vi "target_b2g1.vi"   [LabVIEW 2011]
uses:
  Output - Cluster b2g1.ctl
  Input - Cluster b2g1.ctl
  <vilib>/Platform/TimedLoop/XDataNode/timing_clust.ctl
  <vilib>/Platform/TimedLoop/XDataNode/nitl_modes.ctl
  <vilib>/Platform/TimedLoop/XDataNode/wakeup.ctl
  <vilib>/Platform/TimedLoop/XDataNode/XDataNode.xnode
  <vilib>/Platform/TimedLoop/XDataNode/XDNodeRunTimeDep.lvlib
panel:
  # "The Network Variable Engine and Variable Client Support must be installed on the RT target\nfor this application to function properly. If the Network Variable Engine is not supported on\nthe target (e.g.  FP-2000 with <32MB of RAM), open the project and move the variable library\nto My Computer in the project. Doing this will deploy the variables to localhost but\nwill still require that Variable Client Support be installed on the RT target."
types:
  T1 = typedef "XDNodeRunTimeDep.lvlib/timing_clust.ctl" = cluster{"Expected End [f-1]":u64, "Actual End [f-1]":u64, "Finished Late? [f-1]":bool, "Expected End [i-1]":u64, "Actual End [i-1]":u64, "Finished Late? [i-1]":bool, "Expected Start [i]":u64, "Actual Start [i]":u64, "Expected Start [f]":u64, "Actual Start [f]":u64, "Source Name":string, "Structure Name":string, "Period":i64, "Deadline":i64, "Offset":i64, "Start":i64, "Priority":i32, "Timeout":i32, "Mode":T2, "Wakeup Reason":T3, "Error":errorcluster, "Source Type":string, "Secondary Source Type":string, "Global End Time":u64, "Global Start Time":u64, "Frame Duration":u64, "Iteration Duration":u64, "Assigned CPU":i32, "I/O Scan Engine Mode":u32}
  T2 = typedef "XDNodeRunTimeDep.lvlib/nitl_modes.ctl" = enum32{"No Change", "Process missed periods, maintain original phase", "Discard missed periods, maintain original phase", "Process missed periods, ignore original phase", "Discard missed periods, ignore original phase"}
  T3 = typedef "XDNodeRunTimeDep.lvlib/wakeup.ctl" = enum32{"Normal", "Aborted", "Asynchronous wakeup", "Timing source error", "Timed loop error", "Timeout"}
  T4 = typedef "Output - Cluster b2g1.ctl" = cluster{"DFS-1 [dl]":u64, "FS-3 [l]":dbl, "DFS-1 [l/min]":dbl, "DS-1 [bar]":dbl, "V-10 ZU":bool, "V-14 ZU":bool, "FS-1 [l]":dbl, "FS-2 [l]":dbl, "TS-4 [°C]":dbl, "HS-1":bool, "V-13 [%]":u8, "V-15 [%]":u8, "P-4 [%]":u8, "P-5 [%]":u8, "Dosierung":bool, "MR Max Füllstand":bool, "MR Min Füllstand":bool, "Dosiermenge [l]":sgl, "V-14 AUF":bool, "V-10 AUF":bool, "T-1 Max Füllstand":bool, "T-1 Min Füllstand":bool, "T-2 Max Füllstand":bool, "T-2 Min Füllstand":bool, "pHS-1 [pH]":dbl, "P-4 RUN":bool, "P-5 RUN ":bool, "V-33 AUF":bool, "V-33 ZU":bool, "V-34 AUF":bool, "V-34 ZU":bool, "P-4 ERR":bool, "P-5 ERR":bool, "TS-5 [°C]":dbl, "GZ-1 [dl]":u64, "TS-6 [°C]":dbl, "DS-3 [bar]":dbl, "P-9 RUN":bool}
  T5 = typedef "Input - Cluster b2g1.ctl" = cluster{"V-13 [%]":u8, "V-15 [%]":u8, "Log-Target":bool, "P-4":bool, "P-4 Drehzahl [%]":u8, "Temperaturregelung":bool, "Überdruckregelung":bool, "Füllstandsregulierung":bool, "V-10":bool, "Log-Host":bool, "V-14":bool, "P-5":bool, "P-5 Drehzahl [%]":u8, "HS-1":bool, "Füllstand  P":sgl, "Füllstand I":sgl, "Füllstand D":sgl, "Füllstand Soll [l]":sgl, "Druck  P":sgl, "Druck I":sgl, "Druck D":sgl, "Druck Soll [bar]":sgl, "Temp Soll [°C]":sgl, "Dosierung":bool, "Dosiermenge [l]":sgl, "Dosiergeschw. [l/min]":sgl, "Tank":bool, "Hysterese [°C]":sgl, "MR Füllstandsüberwachung":bool, "Tank Füllstandsüberwachung":bool, "Log Target [ms]":u32, "Log Host [s]":u32, "P-5 EIN [min]":u8, "P-5 AUS [min]":u8, "Zirkulation":bool, "V-33":bool, "V-34":bool, "P-9":bool}
  T6 = cluster{"Durchflussregelung":dbl, "Temperaturregelung":bool, "STOP":bool, "Zirkulation":u64, "Dosierung Zeit":u64}
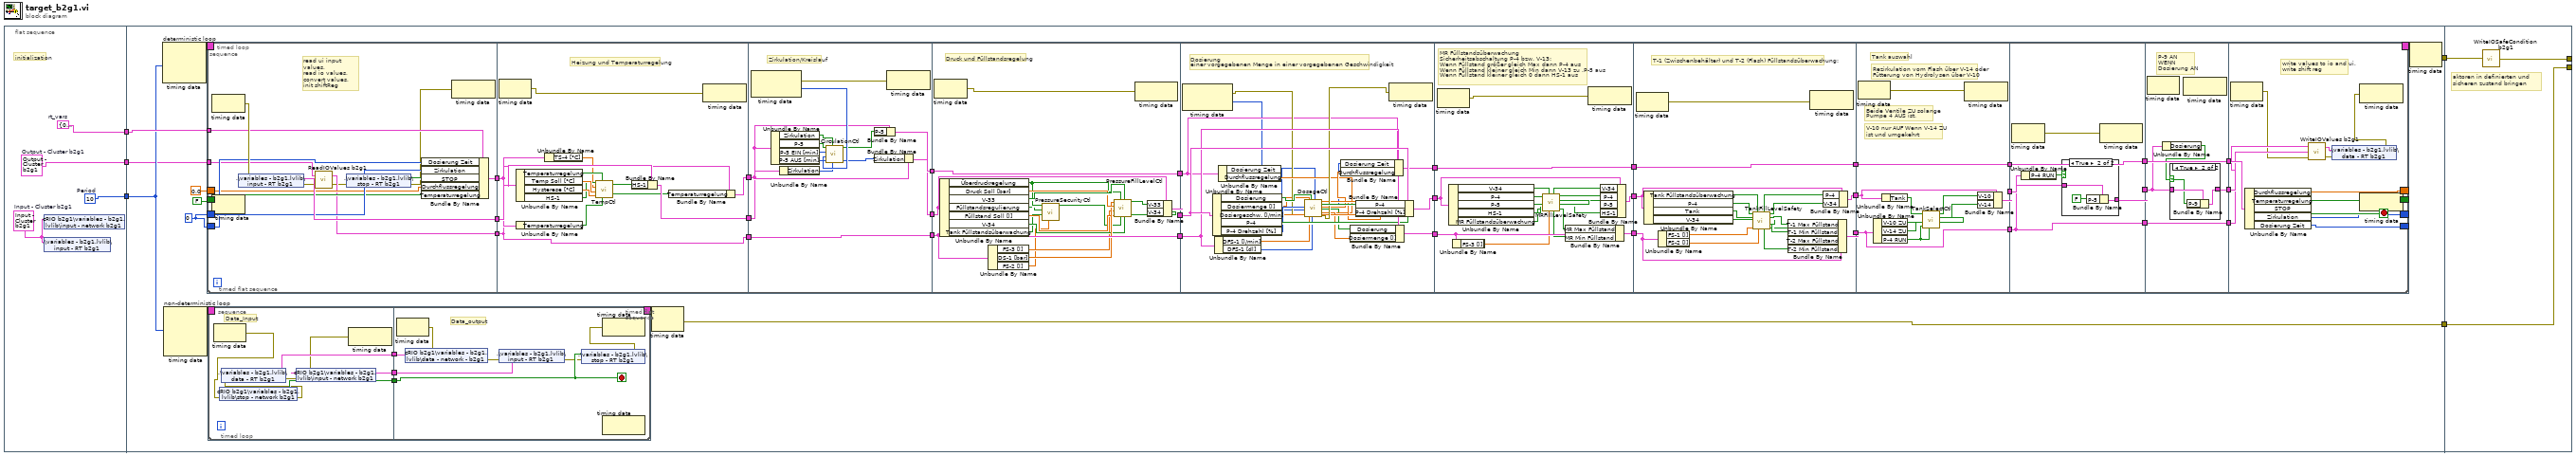
[diagram p0: block diagram]
diagram:
  n1 = flat-sequence {
    tunnel: [w9] -> w5
    tunnel: [w8] -> w4
    tunnel: [w6] -> w3
    tunnel: w5 -> [w15]
    tunnel: w4 -> [w14]
    tunnel: w3 -> [w13]
    tunnel: [w12] -> w2
    tunnel: [w11] -> w1
    tunnel: w2 -> [w329]
    tunnel: w1 -> [w331]
    tunnel: [w330] -> _
    tunnel: [w329] -> _
    frame #0 {
      w6 = T4 {"DFS-1 [dl]"=0, "FS-3 [l]"=0.0, "DFS-1 [l/min]"=0.0, "DS-1 [bar]"=0.0, "V-10 ZU"=FALSE, "V-14 ZU"=FALSE, "FS-1 [l]"=0.0, "FS-2 [l]"=0.0, "TS-4 [°C]"=0.0, "HS-1"=FALSE, "V-13 [%]"=0, "V-15 [%]"=0, "P-4 [%]"=0, "P-5 [%]"=0, "Dosierung"=FALSE, "MR Max Füllstand"=FALSE, "MR Min Füllstand"=FALSE, "Dosiermenge [l]"=0.0, "V-14 AUF"=FALSE, "V-10 AUF"=FALSE, "T-1 Max Füllstand"=FALSE, "T-1 Min Füllstand"=FALSE, "T-2 Max Füllstand"=FALSE, "T-2 Min Füllstand"=FALSE, "pHS-1 [pH]"=0.0, "P-4 RUN"=FALSE, "P-5 RUN "=FALSE, "V-33 AUF"=FALSE, "V-33 ZU"=FALSE, "V-34 AUF"=FALSE, "V-34 ZU"=FALSE, "P-4 ERR"=FALSE, "P-5 ERR"=FALSE, "TS-5 [°C]"=0.0, "GZ-1 [dl]"=0, "TS-6 [°C]"=0.0, "DS-3 [bar]"=0.0, "P-9 RUN"=FALSE}  # Output - Cluster b2g1
      w7 = T5 {"V-13 [%]"=0, "V-15 [%]"=0, "Log-Target"=FALSE, "P-4"=FALSE, "P-4 Drehzahl [%]"=0, "Temperaturregelung"=FALSE, "Überdruckregelung"=FALSE, "Füllstandsregulierung"=FALSE, "V-10"=FALSE, "Log-Host"=FALSE, "V-14"=FALSE, "P-5"=FALSE, "P-5 Drehzahl [%]"=0, "HS-1"=FALSE, "Füllstand  P"=0.0, "Füllstand I"=0.0, "Füllstand D"=0.0, "Füllstand Soll [l]"=0.0, "Druck  P"=0.0, "Druck I"=0.0, "Druck D"=0.0, "Druck Soll [bar]"=0.0, "Temp Soll [°C]"=0.0, "Dosierung"=FALSE, "Dosiermenge [l]"=0.0, "Dosiergeschw. [l/min]"=0.0, "Tank"=FALSE, "Hysterese [°C]"=0.0, "MR Füllstandsüberwachung"=FALSE, "Tank Füllstandsüberwachung"=FALSE, "Log Target [ms]"=0, "Log Host [s]"=0, "P-5 EIN [min]"=0, "P-5 AUS [min]"=0, "Zirkulation"=FALSE, "V-33"=FALSE, "V-34"=FALSE, "P-9"=FALSE}  # Input - Cluster b2g1
      w9 = T6 {"Durchflussregelung"=0.0, "Temperaturregelung"=FALSE, "STOP"=FALSE, "Zirkulation"=0, "Dosierung Zeit"=0}  # rt_vars
      w8 = i64 10  # Period
      # "initialization"
      n2 = shared-variable "cRIO b2g1\\variables - b2g1.lvlib\\input - network b2g1"(w7) -> ()  [unwired: 1 in, 1 out]
      n3 = shared-variable ".\\variables - b2g1.lvlib\\input - RT b2g1"(w7) -> ()  [unwired: 1 in, 1 out]
    }
    frame #1 {
      w10 = u64 0
      n4 = node-c288 ("Input Node")(w14) -> (w21:T1)  [unwired: 2 in]
      n5 = node-c288 ("Input Node")(w14) -> (w19:T1)  [unwired: 3 in]
      n6 = timed-loop "deterministic loop" {
        timing: w21 -> [_]
        timing-out: [_] -> w20
        shift-right: [w65] -> _
        shift-left: 0.0 -> [w64]
        shift-right: [w63] -> _
        shift-left: FALSE ("Temperaturregelung") -> [w61]
        tunnel: w15 -> [w62]
        tunnel: w13 -> [w60]
        shift-right: [w59] -> _
        shift-left: w10 -> [w58]
        shift-right: [w57] -> _
        shift-left: w10 -> [w56]
        stop <- w312 stop-if-true
        n7 = timed-sequence {
          timing: _ -> [_]
          timing-out: _ -> [_]
          tunnel: [w103] -> w65
          tunnel: w64 -> [w102]
          tunnel: [w99] -> w63
          tunnel: w62 -> [w98]
          tunnel: w61 -> [w96]
          tunnel: w60 -> [w91]
          tunnel: [w78] -> w59
          tunnel: w58 -> [w77]
          tunnel: [w73] -> w57
          tunnel: w56 -> [w72]
          n8 = timed-flat-sequence {
            tunnel: [w119] -> w101
            tunnel: [w109] -> w100
            tunnel: w102 -> [w112]
            tunnel: w98 -> [w117]
            tunnel: [w116] -> w97
            tunnel: w96 -> [w111]
            tunnel: w91 -> [w110]
            tunnel: w77 -> [w115]
            tunnel: w72 -> [w114]
            tunnel: w101 -> [w134]
            tunnel: w100 -> [w126]
            tunnel: [w126] -> w84
            tunnel: w97 -> [w130]
            tunnel: [w131] -> w82
            tunnel: [w133] -> w80
            tunnel: w84 -> [w156]
            tunnel: [w156] -> w83
            tunnel: w82 -> [w149]
            tunnel: [w150] -> w81
            tunnel: w80 -> [w147]
            tunnel: [w148] -> w79
            tunnel: [w179] -> w105
            tunnel: w83 -> [w177]
            tunnel: [w177] -> w104
            tunnel: w81 -> [w181]
            tunnel: [w181] -> w95
            tunnel: w79 -> [w178]
            tunnel: w105 -> [w210]
            tunnel: [w208] -> w90
            tunnel: w104 -> [w209]
            tunnel: [w203] -> w89
            tunnel: w95 -> [w195]
            tunnel: [w199] -> w88
            tunnel: w90 -> [w223]
            tunnel: [w222] -> w94
            tunnel: w89 -> [w232]
            tunnel: [w231] -> w93
            tunnel: w88 -> [w234]
            tunnel: [w234] -> w92
            tunnel: w94 -> [w244]
            tunnel: [w245] -> w87
            tunnel: w93 -> [w255]
            tunnel: [w254] -> w86
            tunnel: w92 -> [w257]
            tunnel: [w257] -> w85
            tunnel: w87 -> [w266]
            tunnel: [w267] -> w76
            tunnel: w86 -> [w270]
            tunnel: [w270] -> w75
            tunnel: w85 -> [w273]
            tunnel: [w273] -> w74
            tunnel: w76 -> [w282]
            tunnel: [w281] -> w71
            tunnel: w75 -> [w280]
            tunnel: [w280] -> w69
            tunnel: w74 -> [w284]
            tunnel: [w284] -> w67
            tunnel: w71 -> [w295]
            tunnel: [w296] -> w70
            tunnel: w69 -> [w298]
            tunnel: [w298] -> w68
            tunnel: w67 -> [w297]
            tunnel: [w297] -> w66
            tunnel: w70 -> [w309]
            tunnel: w68 -> [w308]
            tunnel: [w313] -> w103
            tunnel: [w314] -> w99
            tunnel: w66 -> [w315]
            tunnel: [w311] -> w78
            tunnel: [w310] -> w73
            frame #0 {
              # "read ui input values,\nread io values,\nconvert values,\ninit shiftReg"
              n9 = node-c288 ("Output Node")() -> (w118:errorcluster)  [unwired: 1 in]
              n10 = shared-variable ".\\variables - b2g1.lvlib\\input - RT b2g1"(error in=w118) -> (w119:T5, error out=w108:errorcluster)
              n11 = call "ReadIOValues b2g1.vi"("error in"=w108, "Output - Cluster b2g1 2"=w110) -> ("error out"=w107:errorcluster, "Output - Cluster b2g1"=w109:T4)
              n12 = shared-variable ".\\variables - b2g1.lvlib\\stop - RT b2g1"(error in=w107) -> (w113:bool, error out=w106:errorcluster)
              n13 = Bundle By Name(cluster=w117, "Dosierung Zeit"=w114, "Zirkulation"=w115, "STOP"=w113, "Durchflussregelung"=w112, "Temperaturregelung"=w111) -> (w116:T6)
              n14 = node-c288 ("Input Node")(w106) -> ()  [unwired: 1 out]
            }
            frame #1 {
              # "Heizung und Temperaturregelung"
              n15 = node-c288() -> (w138:errorcluster)  [unwired: 1 in]
              n16 = Unbundle By Name(w134) -> ("Temperaturregelung"=w137:bool, "Temp Soll [°C]"=w136:sgl, "Hysterese [°C]"=w135:sgl, "HS-1"=w127:bool)
              n17 = Unbundle By Name(w130) -> ("Temperaturregelung"=w129:bool)
              n18 = Unbundle By Name(w126) -> ("TS-4 [°C]"=w125:dbl)
              n19 = call "TempCtl.vi"("shiftReg"=w129, "enable"=w137, "Hysterese"=w135, "Soll"=w136, "IST"=w125, "heating"=w127) -> ("shiftReg"=w128:bool, "heating"=w132:bool)
              n20 = Bundle By Name(cluster=w134, "HS-1"=w132) -> (w133:T5)
              n21 = Bundle By Name(cluster=w130, "Temperaturregelung"=w128) -> (w131:T6)
              n22 = node-c288(w138) -> ()  [unwired: 1 out]
            }
            frame #2 {
              # "Zirkulation/Kreislauf"
              n23 = node-c288() -> (w157:errorcluster, w155:i64)  [unwired: 1 in]
              n24 = Unbundle By Name(w147) -> ("Zirkulation"=w152:bool, "P-5"=w151:bool, "P-5 EIN [min]"=w154:u8, "P-5 AUS [min]"=w153:u8)
              n25 = Unbundle By Name(w149) -> ("Zirkulation"=w144:u64)
              n26 = call "CirculationCtl.vi"("shiftReg[ms]"=w144, "enable"=w152, "Actual Start [ms]"=w155, "OffTime [min]"=w153, "OnTime [min]"=w154, "Pump"=w151) -> ("shiftReg[ms]"=w145:u64, "Pump"=w146:bool)  [unwired: 3 in, 1 out]
              n27 = Bundle By Name(cluster=w147, "P-5"=w146) -> (w148:T5)
              n28 = Bundle By Name(cluster=w149, "Zirkulation"=w145) -> (w150:T6)
              n29 = node-c288(w157) -> ()  [unwired: 1 out]
            }
            frame #3 {
              # "Druck und Füllstandsregelung"
              n30 = node-c288() -> (w180:errorcluster)  [unwired: 1 in]
              n31 = Unbundle By Name(w178) -> ("Überdruckregelung"=w167:bool, "Druck Soll [bar]"=w175:sgl, "V-33"=w176:bool, "Füllstandsregulierung"=w166:bool, "Füllstand Soll [l]"=w172:sgl, "V-34"=w173:bool, "Tank Füllstandsüberwachung"=w165:bool)
              n32 = Unbundle By Name(w177) -> ("FS-3 [l]"=w171:dbl, "DS-1 [bar]"=w174:dbl, "FS-2 [l]"=w168:dbl)
              n33 = call "PressureSecurityCtl.vi"("FS-2 [l]"=w168, "Tank Füllstandsüberwachung"=w165, "Füllstandsregulierung"=w166, "Überdruckregelung"=w167) -> ("Füllstandsregulierung"=w164:bool)  [unwired: 7 in]
              n34 = call "PressureFillLevelCtl.vi"("LiquidValve"=w173, "GasValve"=w176, "FillLevelCtl"=w164, "PressureCtl"=w167, "V_setpoint"=w172, "V_value"=w171, "P_setpoint"=w175, "P_value"=w174) -> ("LiquidValve"=w169:bool, "GasValve"=w170:bool)  [unwired: 2 in]
              n35 = node-c288(w180) -> ()  [unwired: 1 out]
              n36 = Bundle By Name(cluster=w178, "V-33"=w170, "V-34"=w169) -> (w179:T5)
            }
            frame #4 {
              # "Dosierung \neiner vorgegebenen Menge in einer vorgegebenen Geschwindigkeit"
              n37 = node-c288() -> (w196:errorcluster, w190:i64)  [unwired: 1 in]
              n38 = Unbundle By Name(w210) -> ("Dosierung"=w201:bool, "Dosiermenge [l]"=w187:sgl, "Dosiergeschw. [l/min]"=w204:sgl, "P-4"=w207:bool, "P-4 Drehzahl [%]"=w206:u8)
              n39 = Unbundle By Name(w209) -> ("DFS-1 [l/min]"=w192:dbl, "DFS-1 [dl]"=w193:u64)
              n40 = Unbundle By Name(w195) -> ("Dosierung Zeit"=w191:u64, "Durchflussregelung"=w197:dbl)
              n41 = call "DosageCtl.vi"("setpoint volume flow [l/min]"=w204, "pump"=w207, "value speed [%]"=w206, "shiftReg int"=w191, "shiftReg dbl"=w197, "error in (no error)"=w196, "setpoint volume [l]"=w187, "value volume flow [l/min]"=w192, "enable"=w201, "value volume [dl]"=w193, "Actual Start [f]"=w190) -> ("pump"=w194:bool, "speed [%]"=w202:dbl, "shiftReg int"=w189:u64, "shiftreg dbl"=w198:dbl, "enable"=w188:bool, "volume[l]"=w200:dbl, "error out"=w205:errorcluster)  [unwired: 2 in]
              n42 = Bundle By Name(cluster=w195, "Dosierung Zeit"=w189, "Durchflussregelung"=w198) -> (w199:T6)
              n43 = Bundle By Name(cluster=w209, "Dosierung"=w188, "Dosiermenge [l]"=w200) -> (w203:T4)
              n44 = Bundle By Name(cluster=w210, "P-4"=w194, "P-4 Drehzahl [%]"=w202) -> (w208:T5)
              n45 = node-c288(w205) -> ()  [unwired: 1 out]
            }
            frame #5 {
              # "MR Füllstandsüberwachung\nSicherheitsabschaltung P-4 bzw. V-13:\nWenn Füllstand größer gleich Max dann P-4 aus\nWenn Füllstand kleiner gleich Min dann V-13 zu ,P-5 aus\nWenn Füllstand kleiner gleich 0 dann HS-1 aus"
              n46 = node-c288() -> (w233:errorcluster)  [unwired: 1 in]
              n47 = Unbundle By Name(w223) -> ("V-34"=w227:bool, "P-4"=w226:bool, "P-5"=w225:bool, "HS-1"=w224:bool, "MR Füllstandsüberwachung"=w217:bool)
              n48 = Unbundle By Name(w232) -> ("FS-3 [l]"=w228:dbl)
              n49 = call "MRFillLevelSafety.vi"("fill level [l]"=w228, "Valve"=w227, "enable"=w217, "Heating"=w224, "Circulation"=w225, "Pump"=w226) -> ("max level"=w230:bool, "Heating"=w218:bool, "Circulation"=w219:bool, "Pump"=w220:bool, "min level"=w229:bool, "Valve"=w221:bool)
              n50 = Bundle By Name(cluster=w232, "MR Max Füllstand"=w230, "MR Min Füllstand"=w229) -> (w231:T4)
              n51 = node-c288(w233) -> ()  [unwired: 1 out]
              n52 = Bundle By Name(cluster=w223, "V-34"=w221, "P-4"=w220, "P-5"=w219, "HS-1"=w218) -> (w222:T5)
            }
            frame #6 {
              # "T-1 (Zwischenbehälter) und T-2 (Flash) Füllstandsüberwachung:"
              n53 = node-c288() -> (w256:errorcluster)  [unwired: 1 in]
              n54 = Unbundle By Name(w244) -> ("Tank Füllstandsüberwachung"=w240:bool, "P-4"=w243:bool, "Tank"=w241:bool, "V-34"=w242:bool)
              n55 = Unbundle By Name(w255) -> ("FS-1 [l]"=w249:dbl, "FS-2 [l]"=w251:dbl)
              n56 = call "TankFillLevelSafety.vi"("pump"=w243, "enable"=w240, "tank"=w241, "outlet valve"=w242, "fill level t-1"=w249, "fill level t-2"=w251) -> ("pump"=w247:bool, "outlet valve"=w246:bool, "max level t-1"=w248:bool, "min level t-1"=w253:bool, "min level t-2"=w252:bool, "max level t-2"=w250:bool)  [unwired: 3 in, 1 out]
              n57 = Bundle By Name(cluster=w255, "T-1 Max Füllstand"=w248, "T-1 Min Füllstand"=w253, "T-2 Max Füllstand"=w250, "T-2 Min Füllstand"=w252) -> (w254:T4)
              n58 = node-c288(w256) -> ()  [unwired: 1 out]
              n59 = Bundle By Name(cluster=w244, "P-4"=w247, "V-34"=w246) -> (w245:T5)
            }
            frame #7 {
              # "V-10 nur AUF Wenn V-14 ZU\nist und umgekehrt"
              # "Beide Ventile ZU solange \nPumpe 4 AUS ist."
              # "Rezirkulation vom Flash über V-14 oder \nFütterung von Hydrolysen über V-10"
              # "Tank auswahl"
              n60 = node-c288() -> (w271:errorcluster)  [unwired: 1 in]
              n61 = Unbundle By Name(w270) -> ("V-10 ZU"=w268:bool, "V-14 ZU"=w269:bool, "P-4 RUN"=w263:bool)
              n62 = Unbundle By Name(w266) -> ("Tank"=w272:bool)
              n63 = call "TankSelectCtl.vi"("pump"=w263, "enable"=w263, "valve t-2 close"=w269, "valve t-1 close"=w268, "Tank"=w272) -> ("valve t-2"=w264:bool, "valve t-1"=w265:bool)  [unwired: 5 in]
              n64 = node-c288(w271) -> ()  [unwired: 1 out]
              n65 = Bundle By Name(cluster=w266, "V-10"=w265, "V-14"=w264) -> (w267:T5)
            }
            frame #8 {
              n66 = node-c288() -> (w283:errorcluster)  [unwired: 1 in]
              n67 = Unbundle By Name(w280) -> ("P-4 RUN"=w279:bool)
              n68 = case shown="True" w279 {
                tunnel: w282 -> [w285 w288]
                tunnel: [w285 w287] -> w281
                frame False {
                }
                frame True {
                  n69 = Bundle By Name(cluster=w288, "P-5"=FALSE) -> (w287:T5)
                }
              }
              n70 = node-c288(w283) -> ()  [unwired: 1 out]
            }
            frame #9 {
              # "P-9 AN\nWENN \nDosierung AN"
              n71 = node-c288() -> ()  [unwired: 1 in, 1 out]
              n72 = Unbundle By Name(w295) -> ("Dosierung"=w294:bool)
              n73 = case shown="True" w294 {
                selector: w294 -> [_ w300]
                tunnel: w295 -> [w299 w302]
                tunnel: [w299 w301] -> w296
                frame False {
                }
                frame True {
                  n74 = Bundle By Name(cluster=w302, "P-9"=w300) -> (w301:T5)
                }
              }
              n75 = node-c288() -> ()  [unwired: 1 in, 1 out]
            }
            frame #10 {
              # "write values to io and ui,\nwrite shift reg"
              n76 = node-c288() -> (w306:errorcluster)  [unwired: 1 in]
              n77 = Unbundle By Name(w315) -> ("Durchflussregelung"=w313:dbl, "Temperaturregelung"=w314:bool, "STOP"=w312:bool, "Zirkulation"=w311:u64, "Dosierung Zeit"=w310:u64)
              n78 = call "WriteIOValues b2g1.vi"("error in"=w306, "Output - Cluster b2g1"=w308, "input cluster"=w309) -> ("error out"=w305:errorcluster, "output cluster"=w307:T4)
              n79 = shared-variable ".\\variables - b2g1.lvlib\\data - RT b2g1"(w307, error in=w305) -> (error out=w316:errorcluster)
              n80 = node-c288(w316) -> ()  [unwired: 1 out]
            }
          }
        }
        n81 = node-c288() -> ()  [unwired: 1 in, 1 out]
        n82 = node-c288() -> ()  [unwired: 1 in, 1 out]
      }
      n83 = timed-loop "non-deterministic loop" {
        timing: w19 -> [_]
        timing-out: [_] -> w18
        stop <- w43 stop-if-true
        n84 = timed-sequence {
          timing: _ -> [_]
          timing-out: _ -> [_]
          n85 = timed-flat-sequence {
            tunnel: [w30] -> w24
            tunnel: [w31] -> w23
            tunnel: [w29] -> w22
            tunnel: w24 -> [w43]
            tunnel: w22 -> [w42]
            tunnel: w23 -> [w41]
            frame #0 {
              # "Data_Input"
              n86 = node-c288() -> (w26:errorcluster)  [unwired: 1 in]
              n87 = shared-variable "cRIO b2g1\\variables - b2g1.lvlib\\stop - network b2g1"(error in=w26) -> (w30:bool, error out=w25:errorcluster)
              n88 = shared-variable ".\\variables - b2g1.lvlib\\data - RT b2g1"(error in=w25) -> (w31:T4, error out=w28:errorcluster)
              n89 = shared-variable "cRIO b2g1\\variables - b2g1.lvlib\\input - network b2g1"(error in=w28) -> (w29:T5, error out=w27:errorcluster)
              n90 = node-c288(w27) -> ()  [unwired: 1 out]
            }
            frame #1 {
              # "Data_output"
              n91 = node-c288() -> (w40:errorcluster)  [unwired: 1 in]
              n92 = shared-variable "cRIO b2g1\\variables - b2g1.lvlib\\data - network - b2g1"(w41, error in=w40) -> (error out=w39:errorcluster)
              n93 = shared-variable ".\\variables - b2g1.lvlib\\input - RT b2g1"(w42, error in=w39) -> (error out=w38:errorcluster)
              n94 = shared-variable ".\\variables - b2g1.lvlib\\stop - RT b2g1"(w43, error in=w38) -> (error out=w37:errorcluster)
              n95 = node-c288(w37) -> ()  [unwired: 1 out]
            }
          }
        }
        n96 = node-c288() -> ()  [unwired: 1 in, 1 out]
        n97 = node-c288() -> ()  [unwired: 1 in, 1 out]
      }
      n98 = node-c288 ("Output Node")(w18) -> (w12:errorcluster)
      n99 = node-c288 ("Output Node")(w20) -> (w11:errorcluster)
    }
    frame #2 {
      # "aktoren in definierten und sicheren zustand bringen"
      n100 = call "WriteIOSafeCondition b2g1.vi"("error in"=w331) -> ("error out"=w330:errorcluster)
    }
  }
